vi "_test Duplicate.vi"() -> ()   [LabVIEW 2020]
uses:
  C:/Users/Administrator/Desktop/GIT/Ballard-Arinc-429-XML-Generator/Source/Assemblies/Ballard_Parameter_ni/bin/Debug/Parameters_Arinc429_XML_Tools.dll
  Source/Assemblies/Ballard_Parameter_ni/bin/Debug/Parameters_Arinc429_XML_Tools.dll
  Source/Libraries/Ballard_Parameter_ni/Ballard_Parameter_ni.lvlib
  Source/Libraries/Ballard_Parameter_ni/_tyedefs/parameter_type.ctl
  Source/Libraries/Ballard_Parameter_ni/_tyedefs/label_type.ctl
panel:
  out "SerializeXML":bool
  in  "XML path dup":path
  out "error out":errorcluster
  in  "XML path":path=path "C:/Users/Administrator/Desktop/GIT/Ballard-Arinc-429-XML-Generator/Database Examples/Parameters.xml"
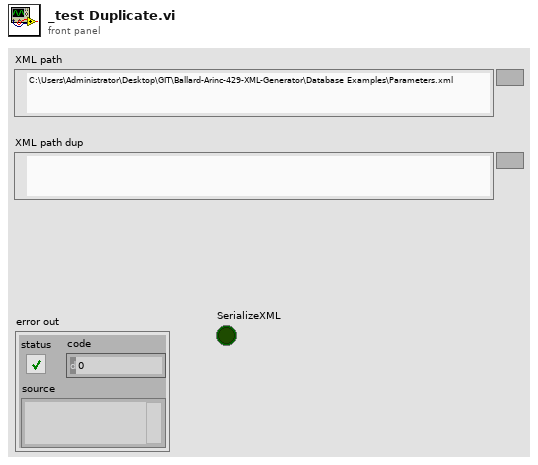
[diagram p1: front panel]
types:
  T1 = typedef "Ballard_Parameter_ni.lvlib/label_type.ctl" = cluster{"createParityChannel":bool, "createSDIChannel":bool, "createSSMChannel":bool, "createTimestampChannel":bool, "labelDecimal":i32, "labelDecimalSpecified":bool, "labelOctal":i32, "labelOctalSpecified":bool, "sdi":i32, "transferType":i32}
  T2 = typedef "Ballard_Parameter_ni.lvlib/parameter_type.ctl" = cluster{"defaultValue":dbl, "encoding":i32, "name":string, "numberOfBits":i32, "offset":dbl, "scale":dbl, "signed":bool, "startBit":i32, "unit":string, "direction":i32}
  T3 = cluster{"channel":i32, "labels":cluster{"Label":T1, "Params":T2[]}[]}
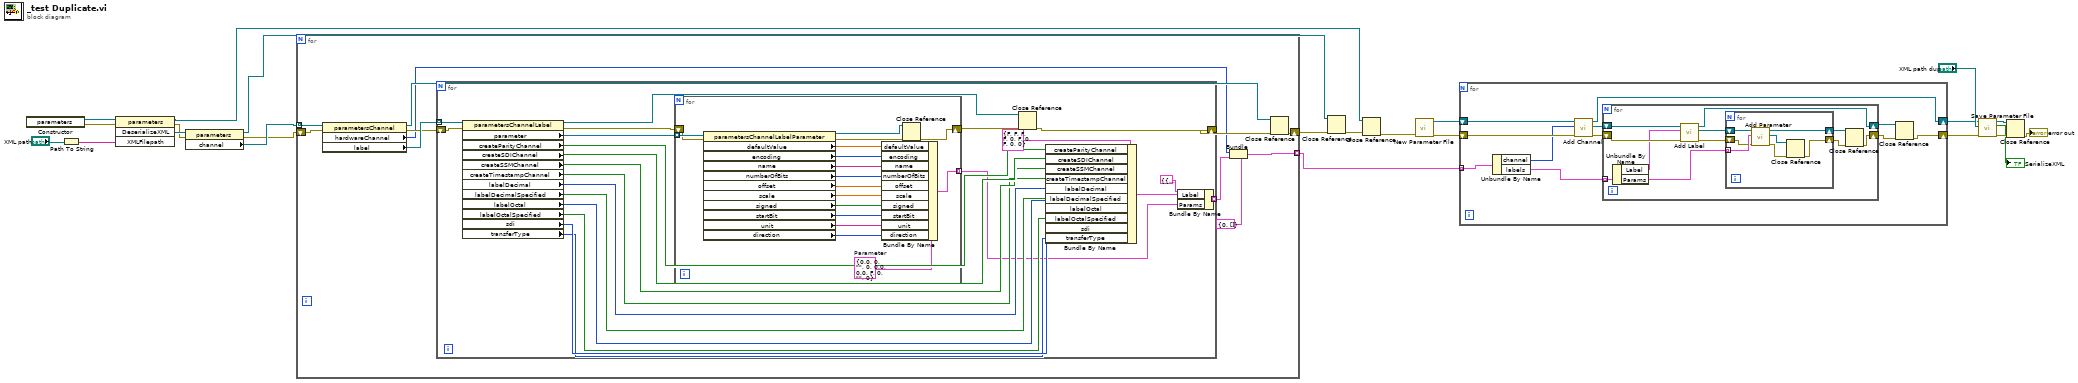
[diagram p0: block diagram]
diagram:
  n1 = constructor class="parameters"() -> (reference out=w23:refnum<k24>, error out=w22:errorcluster)  [unwired: 3 in, 1 out]
  n2 = Path To String(path="XML path") -> (string=w20:string)
  n3 = invoke class="parameters" method="DeserializeXML"(reference=w23, error in=w22, "XMLFilepath"=w20) -> (reference out=w12:refnum<k24>, error out=w18:errorcluster, "DeserializeXML"=w19:refnum<k24>)  [unwired: 1 in, 1 out]
  n4 = property class="parameters"(reference=w19, error in=w18) -> (reference out=w15:refnum<k24>, error out=w16:errorcluster, "channel"=w17:refnum<k24>[])
  n5 = for {
    tunnel: w17 -> [w34] mode=indexing
    shift-right: [w28] -> w14
    shift-left: w16 -> [w33]
    tunnel: [w27] -> w8 mode=indexing
    n6 = property class="parametersChannel"(reference=w34, error in=w33) -> (reference out=w30:refnum<k24>, error out=w31:errorcluster, "hardwareChannel"=w25:i32, "label"=w32:refnum<k24>[])
    n7 = for {
      tunnel: w32 -> [w56] mode=indexing
      shift-right: [w41] -> w29
      shift-left: w31 -> [w55]
      tunnel: [w37] -> w24 mode=indexing
      n8 = property class="parametersChannelLabel"(reference=w56, error in=w55) -> (reference out=w52:refnum<k24>, error out=w54:errorcluster, "parameter"=w53:refnum<k24>[], "createParityChannel"=w50:bool, "createSDIChannel"=w49:bool, "createSSMChannel"=w48:bool, "createTimestampChannel"=w47:bool, "labelDecimal"=w46:i32, "labelDecimalSpecified"=w45:bool, "labelOctal"=w44:i32, "labelOctalSpecified"=w43:bool, "sdi"=w42:i32, "transferType"=w39:i32)
      n9 = for {
        tunnel: w53 -> [w73] mode=indexing
        tunnel: [w62] -> w36 mode=indexing
        shift-right: [w60] -> w51
        shift-left: w54 -> [w72]
        w58 = T2 {"defaultValue"=0.0, "encoding"=0, "name"="", "numberOfBits"=0, "offset"=0.0, "scale"=0.0, "signed"=FALSE, "startBit"=0, "unit"="", "direction"=0}  # Parameter
        n10 = property class="parametersChannelLabelParameter"(reference=w73, error in=w72) -> (reference out=w59:refnum<k24>, error out=w61:errorcluster, "defaultValue"=w71:dbl, "encoding"=w70:i32, "name"=w69:string, "numberOfBits"=w68:i32, "offset"=w67:dbl, "scale"=w66:dbl, "signed"=w65:bool, "startBit"=w64:i32, "unit"=w63:string, "direction"=w57:i32)
        n11 = Bundle By Name(cluster=w58, "defaultValue"=w71, "encoding"=w70, "name"=w69, "numberOfBits"=w68, "offset"=w67, "scale"=w66, "signed"=w65, "startBit"=w64, "unit"=w63, "direction"=w57) -> (w62:T2)
        n12 = Close Reference(reference=w59, error in (no error)=w61) -> (error out=w60:errorcluster)
      }
      n13 = Close Reference(reference=w52, error in (no error)=w51) -> (error out=w41:errorcluster)
      n14 = Bundle By Name(cluster=T1 {"createParityChannel"=FALSE, "createSDIChannel"=FALSE, "createSSMChannel"=FALSE, "createTimestampChannel"=FALSE, "labelDecimal"=0, "labelDecimalSpecified"=FALSE, "labelOctal"=0, "labelOctalSpecified"=FALSE, "sdi"=0, "transferType"=0} ("Label"), "createParityChannel"=w50, "createSDIChannel"=w49, "createSSMChannel"=w48, "createTimestampChannel"=w47, "labelDecimal"=w46, "labelDecimalSpecified"=w45, "labelOctal"=w44, "labelOctalSpecified"=w43, "sdi"=w42, "transferType"=w39) -> (w38:T1)
      n15 = Bundle By Name(cluster=cluster{"Label":T1, "Params":T2[]} {"Label"={"createParityChannel"=FALSE, "createSDIChannel"=FALSE, "createSSMChannel"=FALSE, "createTimestampChannel"=FALSE, "labelDecimal"=0, "labelDecimalSpecified"=FALSE, "labelOctal"=0, "labelOctalSpecified"=FALSE, "sdi"=0, "transferType"=0}, "Params"=[]} ("output cluster"), "Label"=w38, "Params"=w36) -> (w37:cluster{"Label":T1, "Params":T2[]})
    }
    n16 = Bundle(cluster=T3 {"channel"=0, "labels"=[]}, "channel"=w25, "labels"=w24) -> (w27:T3)
    n17 = Close Reference(reference=w30, error in (no error)=w29) -> (error out=w28:errorcluster)
  }
  n18 = Close Reference(reference=w15, error in (no error)=w14) -> (error out=w13:errorcluster)
  n19 = Close Reference(reference=w12, error in (no error)=w13) -> (error out=w11:errorcluster)
  n20 = call "New Parameter File.vi"("error in"=w11) -> ("error out"=w10:errorcluster, "new parameter file"=w9:refnum<k24>)  [unwired: 9 in]
  n21 = for {
    shift-right: [w77] -> w2
    shift-left: w9 -> [w83]
    tunnel: w8 -> [w84] mode=indexing
    shift-right: [w74] -> w7
    shift-left: w10 -> [w82]
    n22 = Unbundle By Name(w84) -> ("channel"=w81:i32, "labels"=w78:cluster{"Label":T1, "Params":T2[]}[])
    n23 = call "Add Channel.vi"("error in"=w82, "hardwareChannel"=w81, "parameter file in"=w83) -> ("error out"=w79:errorcluster, "new channel"=w80:refnum<k24>, "parameter file out"=w77:refnum<k24>)  [unwired: 6 in]
    n24 = for {
      shift-right: [w85] -> w75
      shift-left: w80 -> [w95]
      tunnel: w78 -> [w93] mode=indexing
      shift-right: [w88] -> w76
      shift-left: w79 -> [w94]
      n25 = Unbundle By Name(w93) -> ("Label"=w92:T1, "Params"=w91:T2[])
      n26 = call "Add Label.vi"("error in"=w94, "label configuration"=w92, "channel in"=w95) -> ("error out"=w89:errorcluster, "new label"=w90:refnum<k24>, "channel out"=w85:refnum<k24>)  [unwired: 6 in]
      n27 = for {
        tunnel: w91 -> [w101] mode=indexing
        shift-right: [w99] -> w87
        shift-left: w90 -> [w102]
        shift-right: [w96] -> w86
        shift-left: w89 -> [w100]
        n28 = call "Add Parameter.vi"("error in"=w100, "parameter configuration"=w101, "label in"=w102) -> ("error out"=w98:errorcluster, "new parameter"=w97:refnum<k24>, "label out"=w99:refnum<k24>)  [unwired: 6 in]
        n29 = Close Reference(reference=w97, error in (no error)=w98) -> (error out=w96:errorcluster)
      }
      n30 = Close Reference(reference=w87, error in (no error)=w86) -> (error out=w88:errorcluster)
    }
    n31 = Close Reference(reference=w75, error in (no error)=w76) -> (error out=w74:errorcluster)
  }
  n32 = call "Save Parameter File.vi"("error in"=w7, "XML path"="XML path dup", "parameter file in"=w2) -> ("error out"=w6:errorcluster, "SerializeXML"=→"SerializeXML":bool, "parameter file out"=w4:refnum<k24>)  [unwired: 6 in]
  n33 = Close Reference(reference=w4, error in (no error)=w6) -> (error out=→"error out":errorcluster)
